vi "voltage_measurement.vi"(8 "error in":errorcluster, 10 "Voltage meas settings":T1={"Physical Channel"="Dev1/ai0", "Min Voltage"=-5.0, "Max Voltage"=5.0, "Terminal Configuration"=-1, "Sample Rate"=1000.0, "Number of Samples"=100} {"Terminal Configuration" items=["default"=-1, "RSE"=10083, "NRSE"=10078, "Differential"=10106, "Pseudodifferential"=12529]}) -> (0 "error out":errorcluster, 2 "Waveform Graph":waveform(dbl)[](graph))   [LabVIEW 2024]
uses:
  ctl_voltage_meas_settings_cluster.ctl
  <vilib>/DAQmx/read.llb/DAQmx Read (Analog 1D Wfm NChan NSamp).vi
  <vilib>/DAQmx/create/channels.llb/DAQmx Create Channel (AI-Voltage-Basic).vi
  <vilib>/DAQmx/configure/timing.llb/DAQmx Timing (Sample Clock).vi
  <vilib>/DAQmx/miscellaneous.llb/DAQmx Fill In Error Info.vi
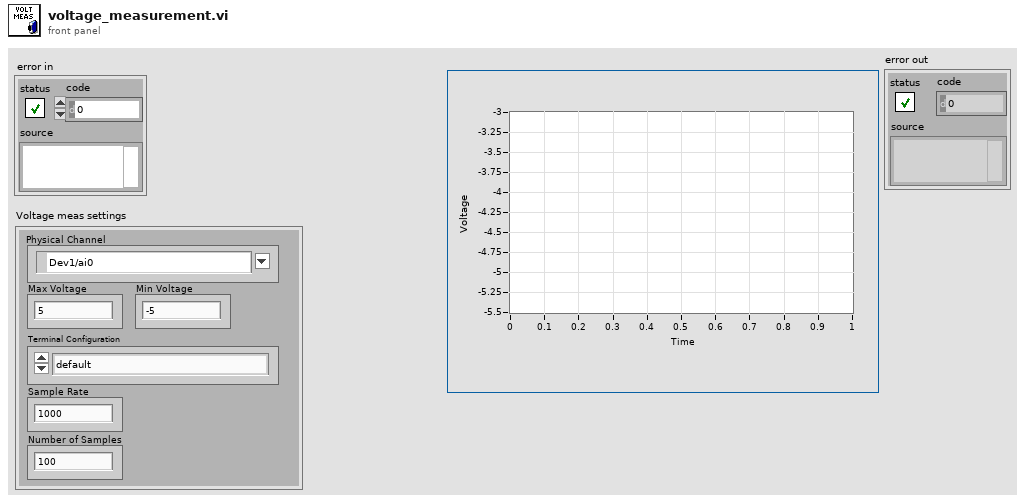
[diagram p1: front panel]
types:
  T1 = typedef "ctl_voltage_meas_settings_cluster.ctl" = cluster{"Physical Channel":tag, "Min Voltage":dbl, "Max Voltage":dbl, "Terminal Configuration":i32, "Sample Rate":dbl, "Number of Samples":i32}
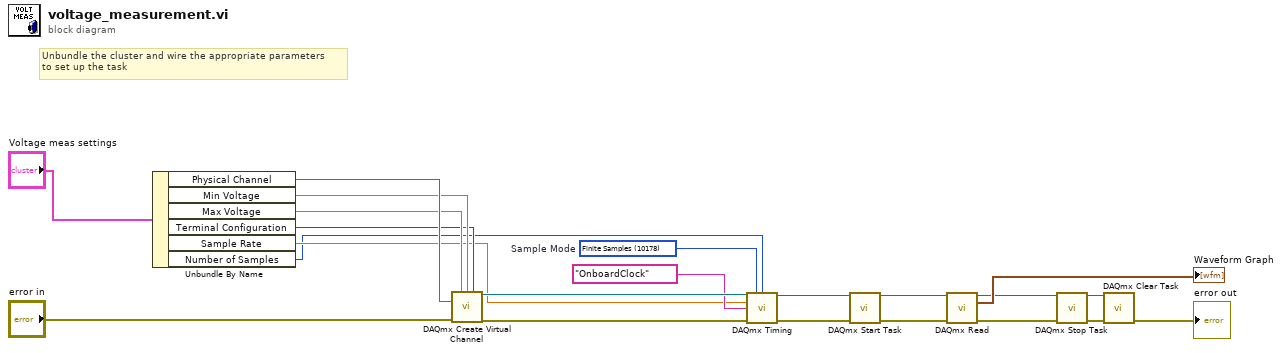
[diagram p0: block diagram]
diagram:
  w22 = 10178 items=["Finite Samples"=10178, "Continuous Samples"=10123, "Hardware Timed Single Point"=12522]  # Sample Mode
  # "Unbundle the cluster and wire the appropriate parameters\nto set up the task"
  n1 = Unbundle By Name("Voltage meas settings") -> ("Physical Channel"=w6:tag, "Min Voltage"=w5:dbl, "Max Voltage"=w4:dbl, "Terminal Configuration"=w3:i32, "Sample Rate"=w2:dbl, "Number of Samples"=w1:i32)
  n2 = call-poly <vilib>:"DAQmx Create Virtual Channel.vi"("maximum value"=w4, "minimum value"=w5, "input terminal configuration"=w3, "physical channels"=w6, "error in"="error in") -> ("task out"=w20:refnum<k21>, "error out"=w21:errorcluster)  [unwired: 9 in]
  n3 = call-poly <vilib>:"DAQmx Timing.vi"("task/channels in"=w20, "sample mode"=w22, "samples per channel"=w1, "rate"=w2, "source"=tag "OnboardClock" ("Sample Clock Source"), "error in"=w21) -> ("task out"=w11:refnum<k21>, "error out"=w10:errorcluster)  [unwired: 8 in]
  n4 = call <vilib>:"DAQmx Start Task.vi"("task/channels in"=w11, "error in"=w10) -> ("task out"=w18:refnum<k21>, "error out"=w17:errorcluster)  [unwired: 12 in]
  n5 = call-poly <vilib>:"DAQmx Read.vi"("task/channels in"=w18, "error in"=w17) -> ("task out"=w13:refnum<k21>, "data"=→"Waveform Graph":waveform(dbl)[], "error out"=w12:errorcluster)  [unwired: 11 in]
  n6 = call <vilib>:"DAQmx Stop Task.vi"("task/channels in"=w13, "error in"=w12) -> ("task out"=w15:refnum<k21>, "error out"=w14:errorcluster)  [unwired: 12 in]
  n7 = call <vilib>:"DAQmx Clear Task.vi"("task in"=w15, "error in"=w14) -> ("error out"=→"error out":errorcluster)  [unwired: 13 in]
